vi "Close_File.vi"(8 "error in (no error)":errorcluster, 11 "Log_Data In":T1) -> (0 "error out":errorcluster, 3 "Log_Data Out":T1)   [LabVIEW 2019, in "Data_Logger.lvlib"]
uses:
  Data_Logger.lvlib
  Logger_Data.ctl
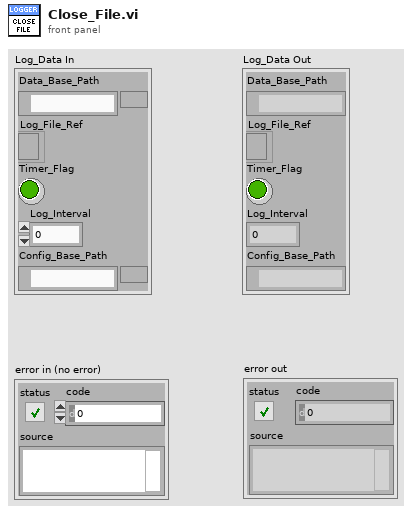
[diagram p1: front panel]
types:
  T1 = typedef "Data_Logger.lvlib/Logger_Data.ctl" = cluster{"Data_Base_Path":path, "Log_File_Ref":refnum<file>, "Timer_Flag":bool, "Log_Interval":dbl, "Config_Base_Path":path}
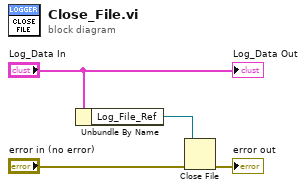
[diagram p0: block diagram]
diagram:
  n1 = Unbundle By Name("Log_Data In") -> ("Log_File_Ref"=w3:refnum<file>)
  n2 = Close File(refnum=w3, error in="error in (no error)") -> (error out=→"error out":errorcluster)  [unwired: 1 out]
  "Log_Data Out" <- "Log_Data In"
